vi "Name FIFOs.vi"(8 "error in (no error)":errorcluster, 10 "Values for Naming":T1={"Bus Number"=1, "Device Number"=1, "Channel Number"=1} {"Channel Number" min=1 step=1; "Device Number" min=1 step=1; "Bus Number" min=1 step=1}, 11 "Communications FIFOs Element":refnum<vi>) -> (0 "error out":errorcluster)   [LabVIEW 2014, in "SPI Engine Scripting.lvlib"]
uses:
  SPI Engine Scripting.lvlib
  State Machine/Controls/Values for Naming.ctl
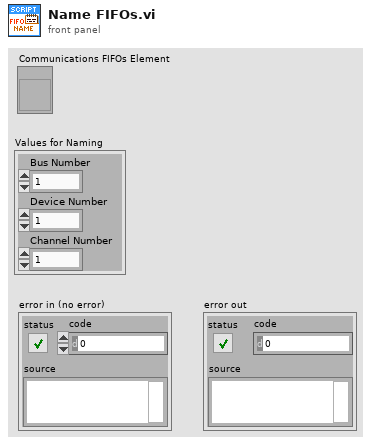
[diagram p1: front panel]
types:
  T1 = typedef "SPI Engine Scripting.lvlib/Values for Naming.ctl" = cluster{"Bus Number":i32, "Device Number":i32, "Channel Number":i32}
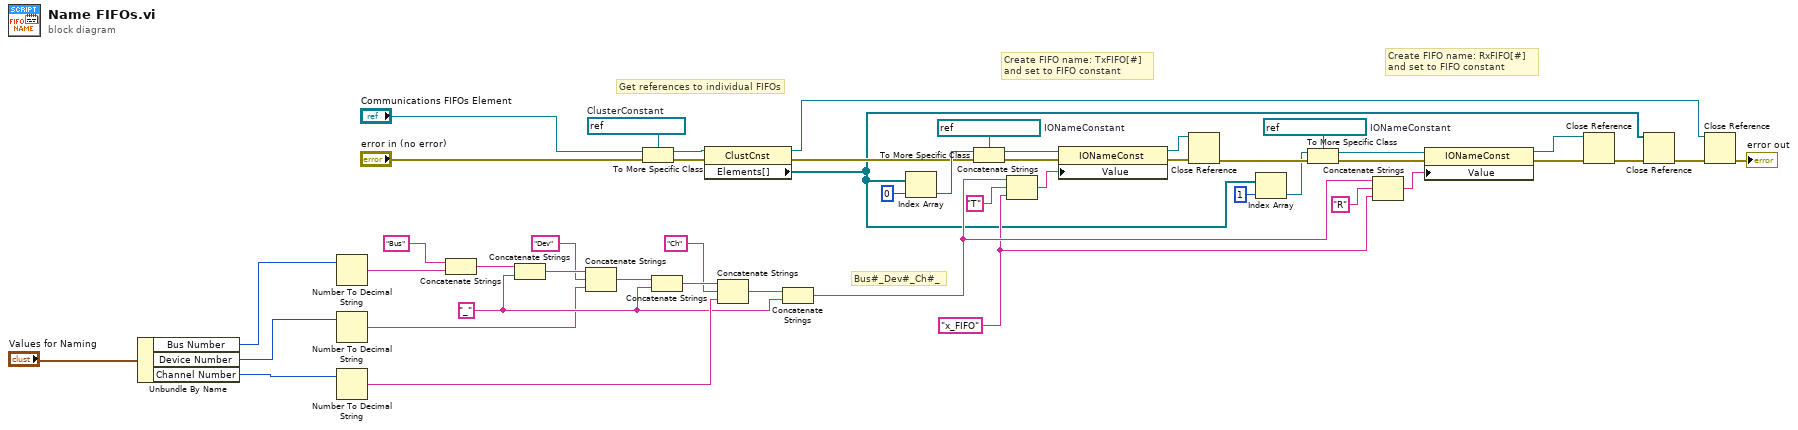
[diagram p0: block diagram]
diagram:
  w10 = "_" ("string")
  w6 = "x_FIFO" ("string")
  w41 = refnum<vi> refnum  # IONameConstant
  w28 = refnum<vi> refnum  # IONameConstant
  w24 = refnum<vi> refnum  # ClusterConstant
  # "Bus#_Dev#_Ch#_"
  # "Create FIFO name: RxFIFO[#]\nand set to FIFO constant"
  # "Create FIFO name: TxFIFO[#]\nand set to FIFO constant"
  # "Get references to individual FIFOs"
  n1 = Unbundle By Name("Values for Naming") -> ("Bus Number"=w19:i32, "Device Number"=w23:i32, "Channel Number"=w22:i32)
  n2 = Number To Decimal String(number=w19) -> (decimal integer string=w9:string)  [unwired: 1 in]
  n3 = Number To Decimal String(number=w23) -> (decimal integer string=w8:string)  [unwired: 1 in]
  n4 = Number To Decimal String(number=w22) -> (decimal integer string=w21:string)  [unwired: 1 in]
  n5 = Concatenate Strings("Bus" ("string"), w9) -> (w17:string)
  n6 = Concatenate Strings(w17, w10) -> (w16:string)
  n7 = Concatenate Strings(w16, "Dev" ("string"), w8) -> (w14:string)
  n8 = To More Specific Class(target class=w24, reference="Communications FIFOs Element", error in="error in (no error)") -> (specific class reference=w26:refnum<vi>, error out=w25:errorcluster)
  n9 = Concatenate Strings(w14, w10) -> (w13:string)
  n10 = property class="ClustCnst"(reference=w26, error in=w25) -> (reference out=w1:refnum<vi>, error out=w29:errorcluster, "Elements[]"=w4:refnum<vi>[])
  n11 = Concatenate Strings(w13, "Ch" ("string"), w21) -> (w11:string)
  n12 = Concatenate Strings(w11, w10) -> (w7:string)
  n13 = Index Array(array=w4, index=0) -> (element=w30:refnum<vi>)
  n14 = To More Specific Class(target class=w28, reference=w30, error in=w29) -> (specific class reference=w32:refnum<vi>, error out=w31:errorcluster)
  n15 = Concatenate Strings(w7, "T" ("string"), w6) -> (w33:string)
  n16 = property class="IONameConst"(reference=w32, error in=w31, "Value"=w33) -> (reference out=w45:refnum<vi>, error out=w44:errorcluster)
  n17 = Close Reference(reference=w45, error in (no error)=w44) -> (error out=w46:errorcluster)
  n18 = Index Array(array=w4, index=1) -> (element=w39:refnum<vi>)
  n19 = To More Specific Class(target class=w41, reference=w39, error in=w46) -> (specific class reference=w37:refnum<vi>, error out=w38:errorcluster)
  n20 = Concatenate Strings(w7, "R" ("string"), w6) -> (w36:string)
  n21 = property class="IONameConst"(reference=w37, error in=w38, "Value"=w36) -> (reference out=w43:refnum<vi>, error out=w42:errorcluster)
  n22 = Close Reference(reference=w43, error in (no error)=w42) -> (error out=w5:errorcluster)
  n23 = Close Reference(reference=w4, error in (no error)=w5) -> (error out=w3:errorcluster)
  n24 = Close Reference(reference=w1, error in (no error)=w3) -> (error out=→"error out":errorcluster)
